vi "init_ccd__secondary_sbig.vi"(0 "Scan Directory":string="Peter_ferguson\\Tcal\\scans\\", 1 "Exposure Time":dbl, 2 "Min nm":dbl, 3 "Max nm":dbl, 4 "Step size":dbl, 6 "Scan_prefix":string) -> (5 "Working Directory":path)   [LabVIEW 2018]
uses:
  <vilib>/Utility/sysdir.llb/System Directory Type.ctl
panel:
  in  "Name of CCD control code":string="CCDautomation_prefix.exe"
  in  "Password":string="astrolabtywin"
  in  "Username":string="astrolab\\astrolab"
  in  "IP address":string="165.91.221.116"
  out "substring":string
  in  "Boolean":bool=TRUE
  out "Commands Sent":string
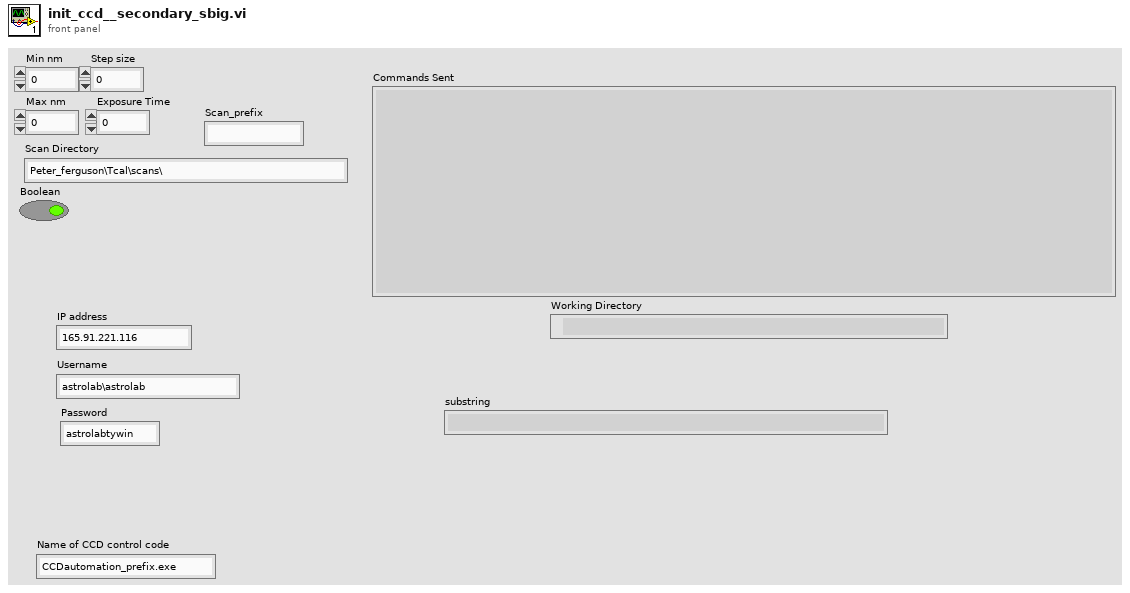
[diagram p1: front panel]
types:
  T1 = enum16{"open", "replace", "create", "open or create", "replace or create", "replace or create with confirmation"}
  T2 = typedef "System Directory Type.ctl" = i32
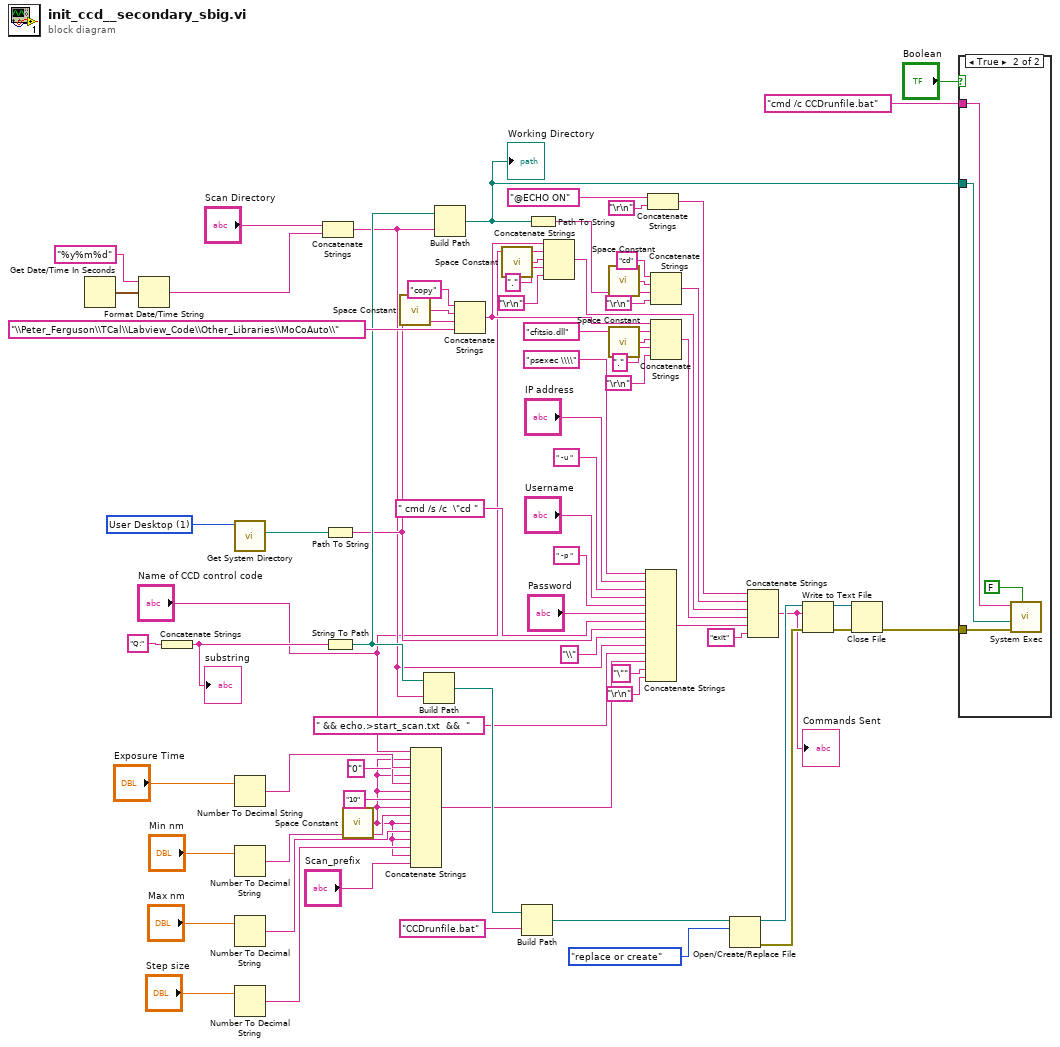
[diagram p0: block diagram]
diagram:
  w70 = T2 1 items=["User Home"=0, "User Desktop"=1, "User Documents"=2, "User Application Data"=3, "User Preferences"=4, "User Temporary"=5, "Public Documents"=6, "Public Application Data"=7, "Public Preferences"=8, "Public Cache"=13, "System Core Libraries"=9, "System Installed Libraries"=10, "Application Files"=11, "Boot Volume Root"=12] ("system directory type")
  n1 = Get Date/Time In Seconds() -> (seconds since 1Jan1904=w72:timestamp)
  n2 = Format Date/Time String(time format string (%c)="%y%m%d", seconds (now)=w72) -> (date/time string=w68:string)  [unwired: 1 in]
  n3 = Concatenate Strings("Q:" ("string")) -> (w23:string)
  "substring" <- w23
  n4 = call <vilib>:"Get System Directory.vi"("system directory type"=w70) -> ("system directory"=w22:path)  [unwired: 10 in]
  n5 = Number To Decimal String(number="Exposure Time") -> (decimal integer string=w45:string)  [unwired: 1 in]
  n6 = Number To Decimal String(number="Min nm") -> (decimal integer string=w28:string)  [unwired: 1 in]
  n7 = Number To Decimal String(number="Max nm") -> (decimal integer string=w27:string)  [unwired: 1 in]
  n8 = Number To Decimal String(number="Step size") -> (decimal integer string=w26:string)  [unwired: 1 in]
  n9 = Concatenate Strings("Scan Directory", w68) -> (w8:string)
  n10 = Path To String(path=w22) -> (string=w10:string)
  n11 = String To Path(string=w23) -> (path=w20:path)
  n12 = call <vilib>:"Space Constant.vi"() -> ("String"=w2:string)
  n13 = call <vilib>:"Space Constant.vi"() -> ("String"=w60:string)
  n14 = Concatenate Strings("Name of CCD control code", w2, w45, w2, "0" ("string"), w2, "10" ("string"), w2, w28, w2, w27, w2, w26, w2, "Scan_prefix") -> (w4:string)
  n15 = Build Path(base path=w20, name or relative path=w8) -> (appended path=w11:path)
  n16 = Build Path(base path=w20, name or relative path=w8) -> (appended path=w21:path)
  "Working Directory" <- w21
  n17 = Concatenate Strings("copy", w60, w10, "\\Peter_Ferguson\\TCal\\Labview_Code\\Other_Libraries\\MoCoAuto\\" ("string")) -> (w52:string)
  n18 = call <vilib>:"Space Constant.vi"() -> ("String"=w56:string)
  n19 = Build Path(base path=w11, name or relative path="CCDrunfile.bat") -> (appended path=w39:path)
  n20 = Path To String(path=w21) -> (string=w63:string)
  n21 = Concatenate Strings(w52, "Name of CCD control code", w56, "." ("string"), "\r\n") -> (w53:string)
  n22 = call <vilib>:"Space Constant.vi"() -> ("String"=w64:string)
  n23 = call <vilib>:"Space Constant.vi"() -> ("String"=w50:string)
  n24 = Concatenate Strings("psexec \\\\" ("string"), "IP address", " -u " ("string"), "Username", " -p " ("string"), "Password", " cmd /s /c  \"cd " ("string"), w10, "\\" ("string"), w8, " && echo.>start_scan.txt  &&  " ("string"), w4, "\"" ("string"), "\r\n") -> (w12:string)
  n25 = Concatenate Strings("@ECHO ON" ("string"), "\r\n") -> (w58:string)
  n26 = Concatenate Strings("cd" ("string"), w64, w63, "\r\n") -> (w57:string)
  n27 = Concatenate Strings(w52, "cfitsio.dll" ("string"), w50, "." ("string"), "\r\n") -> (w47:string)
  n28 = Open/Create/Replace File(file path (use dialog)=w39, operation (0:open)=T1."replace or create") -> (refnum out=w36:refnum<file>, error out=w35:errorcluster)  [unwired: 4 in, 1 out]
  n29 = Concatenate Strings(w58, w57, w53, w47, w12, "exit" ("string")) -> (w33:string)
  "Commands Sent" <- w33
  n30 = Write to Text File(file (use dialog)=w36, text=w33, error in=w35) -> (refnum out=w37:refnum<file>, error out=w34:errorcluster)  [unwired: 1 in, 1 out]
  n31 = Close File(refnum=w37, error in=w34) -> (error out=w31:errorcluster)  [unwired: 1 out]
  n32 = case shown="True" "Boolean" {
    tunnel: w21 -> [_ w76]
    tunnel: "cmd /c CCDrunfile.bat" ("command line") -> [_ w75]
    tunnel: w31 -> [_ w73]
    frame False {
    }
    frame True {
      n33 = call <vilib>:"System Exec.vi"("wait until completion? (T)"=FALSE, "error in (no error)"=w73, "working directory"=w76, "command line"=w75) -> ()  [unwired: 4 in, 4 out]
    }
  }
